vi "Configure Spurious Emission (Measurement Setup).vi"(0 "VISA resource name":refnum<visa-resource-name>, 1 "Spurious Segment Mode (0:Auto)":i32(ring) items=["Auto", "Manual"], 2 "Spurious Summary Table (0:Range)":i32(ring) items=["Range", "Result"], 3 "Enable Low Phase  Noise (F:Disable)":bool, 5 "Spurious Fail Stop Mode (1:On)":i32(ring)=1 items=["Off", "On"], 7 "Spurious Result Type (0:Worst)":i32(ring) items=["Worst", "Exam", "Peak", "Full"], 9 "Spurious Summary Page Auto Numbering (1:On)":i32(ring)=1 items=["Off", "On"], 11 "error in (no error)":errorcluster, 12 "Spurious Time Domain Mode (1:On)":i32(ring)=1 items=["Off", "On"]) -> (4 "VISA resource name out":refnum<visa-resource-name>, 15 "error out":errorcluster)   [LabVIEW 2020, in "Anritsu Signal Analyzer Series.lvlib"]
doc: "Configures the Spurious Emission measurement parameters."
uses:
  Anritsu Signal Analyzer Series.lvlib
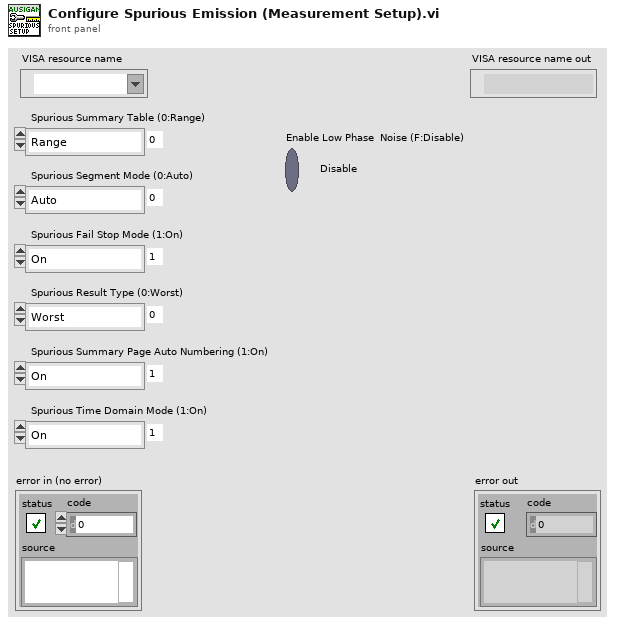
[diagram p1: front panel]
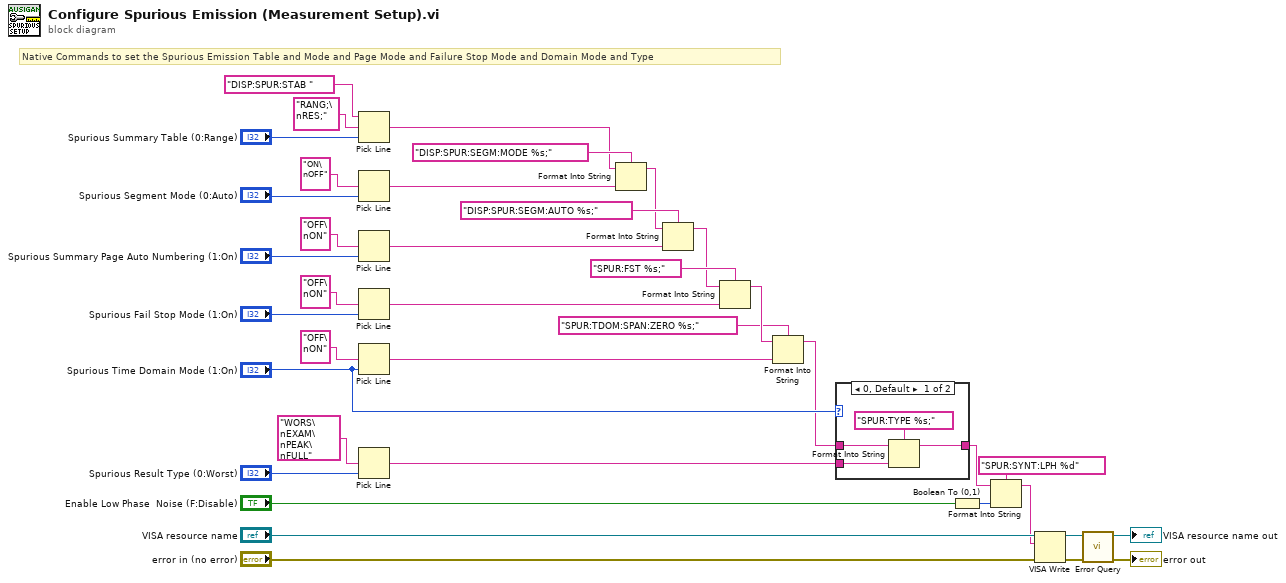
[diagram p0: block diagram]
diagram:
  # "Native Commands to set the Spurious Emission Table and Mode and Page Mode and Failure Stop Mode and Domain Mode and Type"
  n1 = Pick Line(string ("")="DISP:SPUR:STAB " ("_CommandSet"), multi-line string="RANG;\nRES;" ("複数行文字列"), line index="Spurious Summary Table (0:Range)") -> (output string=w9:string)
  n2 = Pick Line(multi-line string="ON\nOFF" ("複数行文字列"), line index="Spurious Segment Mode (0:Auto)") -> (output string=w18:string)  [unwired: 1 in]
  n3 = Pick Line(multi-line string="OFF\nON" ("複数行文字列"), line index="Spurious Summary Page Auto Numbering (1:On)") -> (output string=w14:string)  [unwired: 1 in]
  n4 = Pick Line(multi-line string="OFF\nON" ("複数行文字列"), line index="Spurious Fail Stop Mode (1:On)") -> (output string=w13:string)  [unwired: 1 in]
  n5 = Pick Line(multi-line string="OFF\nON" ("複数行文字列"), line index="Spurious Time Domain Mode (1:On)") -> (output string=w12:string)  [unwired: 1 in]
  n6 = Pick Line(multi-line string="WORS\nEXAM\nPEAK\nFULL" ("複数行文字列"), line index="Spurious Result Type (0:Worst)") -> (output string=w7:string)  [unwired: 1 in]
  n7 = Format Into String(format string="DISP:SPUR:SEGM:MODE %s;" ("_CommandSet"), initial string=w9, w18) -> (resulting string=w21:string)  [unwired: 1 in, 1 out]
  n8 = Format Into String(format string="DISP:SPUR:SEGM:AUTO %s;" ("_CommandSet"), initial string=w21, w14) -> (resulting string=w20:string)  [unwired: 1 in, 1 out]
  n9 = Format Into String(format string="SPUR:FST %s;" ("_CommandSet"), initial string=w20, w13) -> (resulting string=w24:string)  [unwired: 1 in, 1 out]
  n10 = Format Into String(format string="SPUR:TDOM:SPAN:ZERO %s;" ("_CommandSet"), initial string=w24, w12) -> (resulting string=w2:string)  [unwired: 1 in, 1 out]
  n11 = case shown="0, Default" "Spurious Time Domain Mode (1:On)" {
    tunnel: w7 -> [w42 _]
    tunnel: w2 -> [w41 w43]
    tunnel: [w39 w43] -> w3
    frame 0, Default {
      n12 = Format Into String(format string="SPUR:TYPE %s;" ("_CommandSet"), initial string=w41, w42) -> (resulting string=w39:string)  [unwired: 1 in, 1 out]
    }
    frame 1 {
    }
  }
  n13 = Boolean To (0,1)(Boolean="Enable Low Phase  Noise (F:Disable)") -> (0, 1=w4:i16)
  n14 = Format Into String(format string="SPUR:SYNT:LPH %d", initial string=w3, w4) -> (resulting string=w1:string)  [unwired: 1 in, 1 out]
  n15 = VISA Write(VISA resource name="VISA resource name", write buffer=w1, error in (no error)="error in (no error)") -> (VISA resource name out=w28:refnum<visa-resource-name>, error out=w27:errorcluster)  [unwired: 1 out]
  n16 = call "Error Query.vi"("error in (no error)"=w27, "VISA resource name"=w28) -> ("error out"=→"error out":errorcluster, "VISA resource name out"=→"VISA resource name out":refnum<visa-resource-name>)  [unwired: 6 in, 2 out]
